vi "CFTS-Find Available Acoustic Systems.vi"() -> (2 "Acoustic Systems":string[](array[string]))   [LabVIEW 2020]
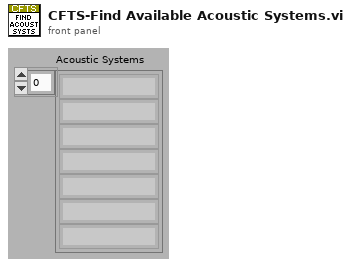
[diagram p1: front panel]
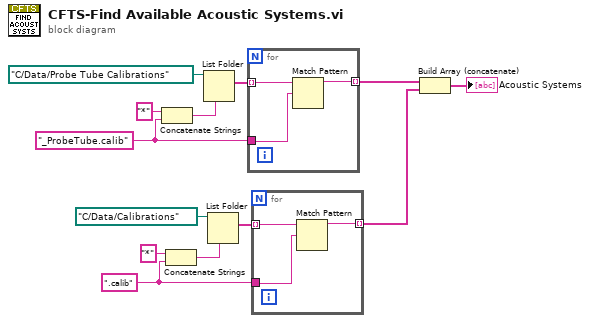
[diagram p0: block diagram]
diagram:
  w4 = ".calib" ("string")
  w10 = "_ProbeTube.calib" ("string")
  n1 = Concatenate Strings("*" ("string"), w10) -> (w11:string)
  n2 = Concatenate Strings("*" ("string"), w4) -> (w5:string)
  n3 = List Folder(path=path "C:/Data/Probe Tube Calibrations", pattern=w11) -> (filenames=w12:string[])  [unwired: 2 in, 3 out]
  n4 = List Folder(path=path "C:/Data/Calibrations", pattern=w5) -> (filenames=w6:string[])  [unwired: 2 in, 3 out]
  n5 = for {
    tunnel: w12 -> [w16] mode=indexing
    tunnel: w10 -> [w15]
    tunnel: [w14] -> w8 mode=indexing
    n6 = Match Pattern(string=w16, regular expression=w15) -> (before substring=w14:string)  [unwired: 1 in, 3 out]
  }
  n7 = for {
    tunnel: w6 -> [w19] mode=indexing
    tunnel: w4 -> [w18]
    tunnel: [w17] -> w1 mode=indexing
    n8 = Match Pattern(string=w19, regular expression=w18) -> (before substring=w17:string)  [unwired: 1 in, 3 out]
  }
  n9 = Build Array (concatenate)(w8, w1) -> (→"Acoustic Systems":string[])
